vi "Auto Align.vi"(4 "sign":dbl) -> (0 "y-axis":dbl, 1 "x-axis":dbl)   [LabVIEW 2012]
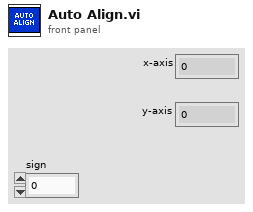
[diagram p1: front panel]
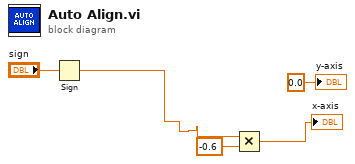
[diagram p0: block diagram]
diagram:
  n1 = Sign(1:"sign") -> (0:w2:dbl)
  n2 = Multiply(x=w2, y=-0.6) -> (x*y=→"x-axis":dbl)
  "y-axis" <- 0.0 ("y-axis")
